vi "Test Compression.vi"() -> ()   [LabVIEW 2015, in "LSR Transmission.lvlib"]
uses:
  LSR Transmission.lvlib
panel:
  out "Ratio":dbl
  out "Decompressed string":string
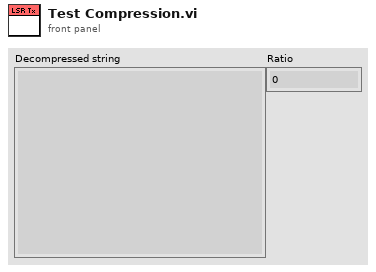
[diagram p1: front panel]
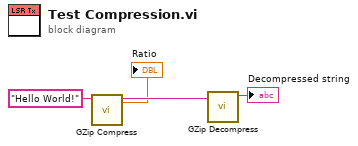
[diagram p0: block diagram]
diagram:
  n1 = call "GZip Compress.vi"("Uncompressed string"="Hello World!") -> ("GZip compressed string"=w4:string, "Ratio"=→"Ratio":dbl)  [unwired: 8 in, 1 out]
  n2 = call "GZip Decompress.vi"("GZip compressed string"=w4) -> ("Decompressed string"=→"Decompressed string":string)  [unwired: 9 in, 1 out]
